vi "副屏设置.vi"() -> ()   [LabVIEW 2016, in "副屏.lvlib"]
uses:
  <vilib>/Utility/config.llb/NI_LVConfig.lvlib
panel:
  in  "启用副屏":bool=TRUE caption="氨氮禁用"
  in  "关闭":bool
  in  "底部状态栏显示信息":string="一体化微型水质监测系统"
  in  "流速":bool caption="氨氮禁用"
  in  "瞬时流量":bool caption="氨氮禁用"
  in  "湿度":bool=TRUE caption="氨氮禁用"
  in  "水位":bool caption="氨氮禁用"
  in  "室温":bool=TRUE caption="氨氮禁用"
  in  "CODCr":bool caption="氨氮禁用"
  in  "CODMn":bool caption="氨氮禁用"
  in  "总氮":bool caption="氨氮禁用"
  in  "总磷":bool caption="氨氮禁用"
  in  "氨氮":bool caption="氨氮禁用"
  in  "Turb":bool caption="氨氮禁用"
  in  "Cond":bool caption="氨氮禁用"
  in  "DO":bool caption="氨氮禁用"
  in  "pH":bool caption="氨氮禁用"
  in  "水温":bool caption="氨氮禁用"
  # "副屏显示信息设置"
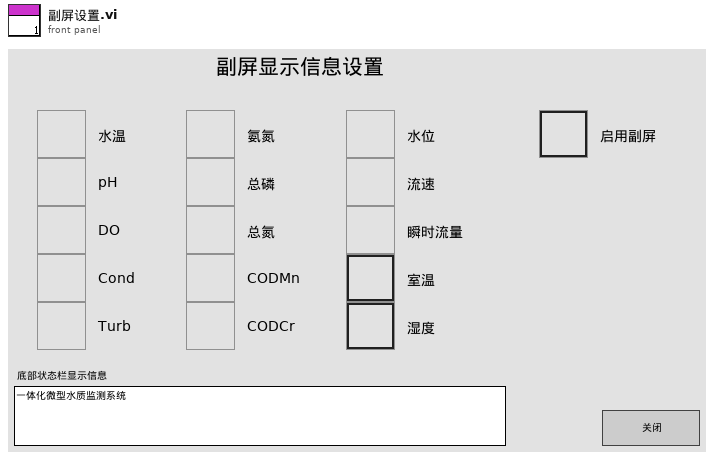
[diagram p1: front panel]
types:
  T1 = typedef "NI_LVConfig.lvlib/Config Data RefNum.ctl" = refnum<k1>
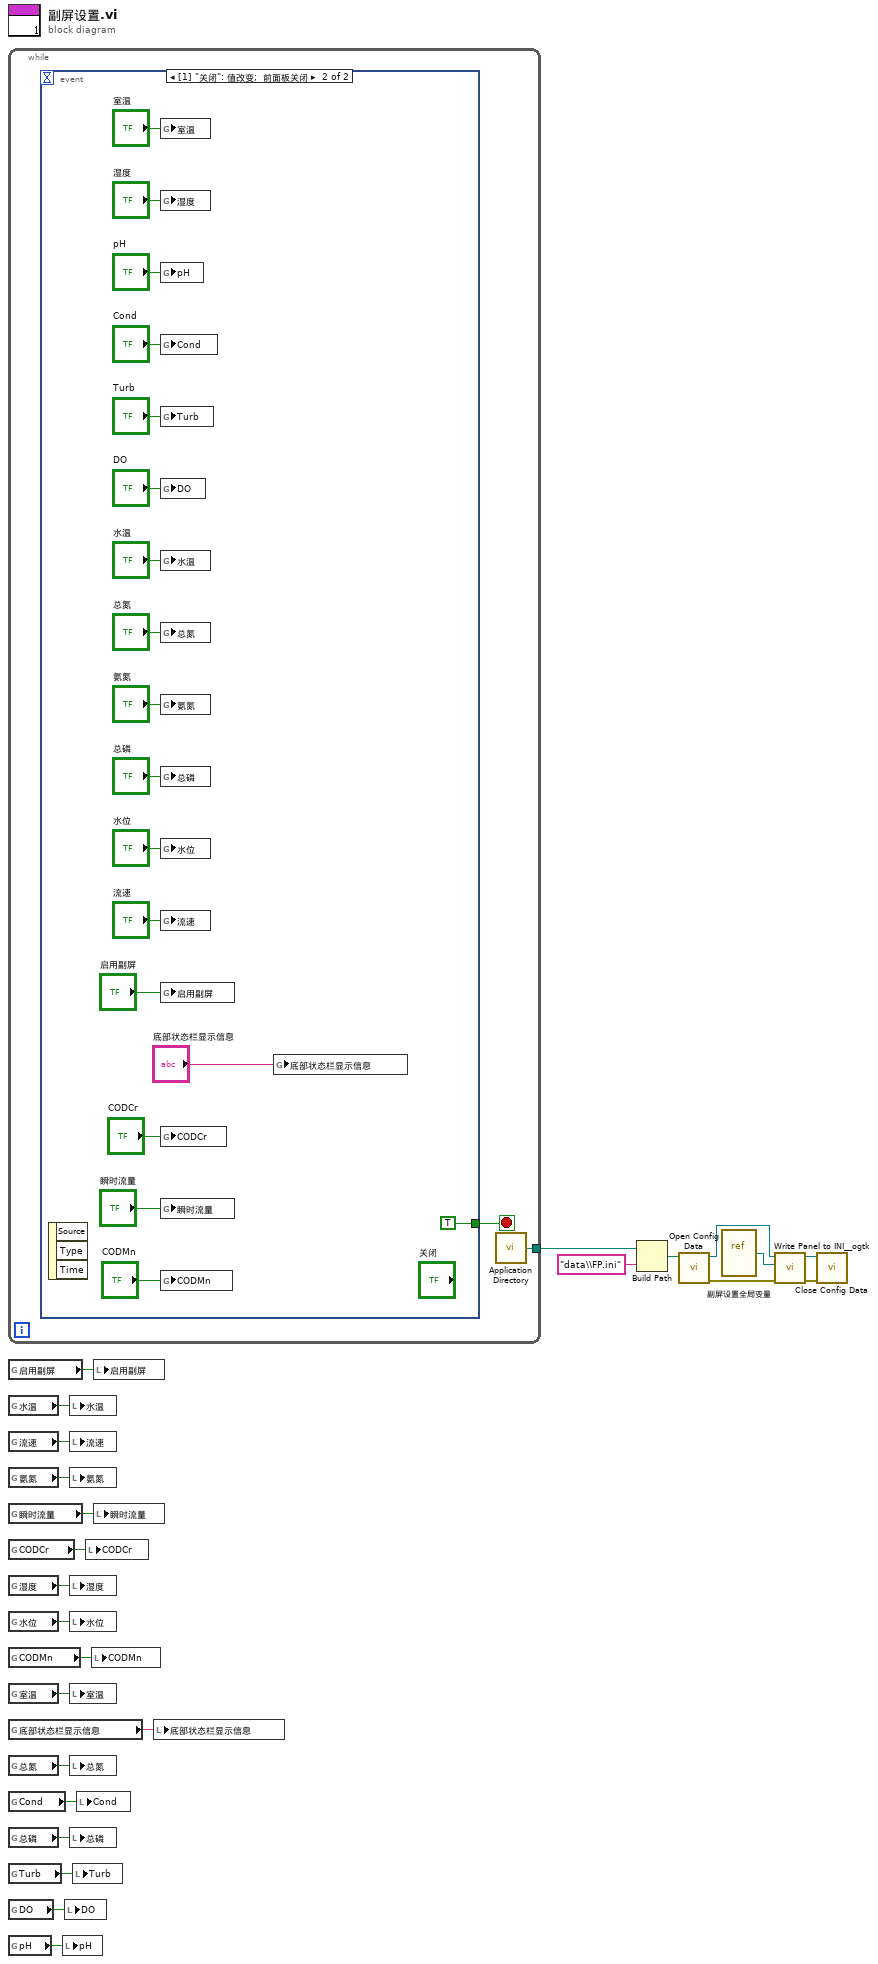
[diagram p0: block diagram]
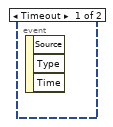
[diagram p2: hidden frame]
diagram:
  n1 = while {
    tunnel: [w26] -> w2
    stop <- w27 stop-if-true
    n2 = event shown="[1] \"关闭\": 值改变;  前面板关闭" {
      selector: _ -> [_ _]
      dyn-events: _ -> [_ _]
      timeout: _ -> [_ _]
      tunnel: [_ TRUE] -> w27
      event Timeout {
        n3 = event-data() -> ()  [unwired: 1 in, 3 out]
      }
      event "关闭": Value Change; Panel Close {
        n4 = event-data() -> ()  [unwired: 1 in, 3 out]
        n5 = global write "副屏设置全局变量.vi" "室温"("室温") -> ()
        n6 = global write "副屏设置全局变量.vi" "湿度"("湿度") -> ()
        n7 = global write "副屏设置全局变量.vi" "pH"("pH") -> ()
        n8 = global write "副屏设置全局变量.vi" "Cond"("Cond") -> ()
        n9 = global write "副屏设置全局变量.vi" "Turb"("Turb") -> ()
        n10 = global write "副屏设置全局变量.vi" "DO"("DO") -> ()
        n11 = global write "副屏设置全局变量.vi" "水温"("水温") -> ()
        n12 = global write "副屏设置全局变量.vi" "总氮"("总氮") -> ()
        n13 = global write "副屏设置全局变量.vi" "氨氮"("氨氮") -> ()
        n14 = global write "副屏设置全局变量.vi" "总磷"("总磷") -> ()
        n15 = global write "副屏设置全局变量.vi" "水位"("水位") -> ()
        n16 = global write "副屏设置全局变量.vi" "流速"("流速") -> ()
        n17 = global write "副屏设置全局变量.vi" "启用副屏"("启用副屏") -> ()
        n18 = global write "副屏设置全局变量.vi" "CODCr"("CODCr") -> ()
        n19 = global write "副屏设置全局变量.vi" "瞬时流量"("瞬时流量") -> ()
        n20 = global write "副屏设置全局变量.vi" "CODMn"("CODMn") -> ()
        n21 = global write "副屏设置全局变量.vi" "底部状态栏显示信息"("底部状态栏显示信息") -> ()
      }
    }
    n22 = call <vilib>:"Application Directory.vi"() -> ("Application Directory"=w26:path)
  }
  n23 = global read "副屏设置全局变量.vi" "启用副屏"() -> (w1:bool)
  n24 = global read "副屏设置全局变量.vi" "水温"() -> (w25:bool)
  n25 = global read "副屏设置全局变量.vi" "流速"() -> (w19:bool)
  n26 = global read "副屏设置全局变量.vi" "氨氮"() -> (w24:bool)
  n27 = global read "副屏设置全局变量.vi" "瞬时流量"() -> (w17:bool)
  n28 = global read "副屏设置全局变量.vi" "CODCr"() -> (w23:bool)
  n29 = global read "副屏设置全局变量.vi" "湿度"() -> (w16:bool)
  n30 = global read "副屏设置全局变量.vi" "水位"() -> (w22:bool)
  n31 = global read "副屏设置全局变量.vi" "CODMn"() -> (w21:bool)
  n32 = global read "副屏设置全局变量.vi" "室温"() -> (w13:bool)
  n33 = global read "副屏设置全局变量.vi" "底部状态栏显示信息"() -> (w20:string)
  n34 = global read "副屏设置全局变量.vi" "总氮"() -> (w14:bool)
  n35 = global read "副屏设置全局变量.vi" "Cond"() -> (w18:bool)
  n36 = global read "副屏设置全局变量.vi" "总磷"() -> (w11:bool)
  n37 = global read "副屏设置全局变量.vi" "Turb"() -> (w12:bool)
  n38 = global read "副屏设置全局变量.vi" "DO"() -> (w15:bool)
  n39 = global read "副屏设置全局变量.vi" "pH"() -> (w10:bool)
  n40 = local write "pH"(w10) -> ()
  n41 = local write "DO"(w15) -> ()
  n42 = local write "水温"(w25) -> ()
  n43 = local write "流速"(w19) -> ()
  n44 = local write "氨氮"(w24) -> ()
  n45 = local write "湿度"(w16) -> ()
  n46 = local write "水位"(w22) -> ()
  n47 = local write "室温"(w13) -> ()
  n48 = local write "总氮"(w14) -> ()
  n49 = local write "总磷"(w11) -> ()
  n50 = local write "Turb"(w12) -> ()
  n51 = local write "Cond"(w18) -> ()
  n52 = local write "CODCr"(w23) -> ()
  n53 = local write "CODMn"(w21) -> ()
  n54 = local write "启用副屏"(w1) -> ()
  n55 = local write "瞬时流量"(w17) -> ()
  n56 = local write "底部状态栏显示信息"(w20) -> ()
  n57 = Build Path(base path=w2, name or relative path="data\\FP.ini" ("名称或相对路径")) -> (appended path=w4:path)
  n58 = call <vilib>:"Open Config Data.vi"("configuration file path"=w4) -> ("error out"=w8:errorcluster, "refnum"=w5:T1)  [unwired: 8 in, 1 out]
  n59 = vi-ref "副屏设置全局变量.vi"() -> (w6:refnum<vi>)
  n60 = call <userlib>:"Write Panel to INI__ogtk.vi"("error in (no error)"=w8, "VI ref"=w6, "refnum"=w5) -> ("error out"=w9:errorcluster, "refnum out"=w7:T1)  [unwired: 7 in]
  n61 = call <vilib>:"Close Config Data.vi"("error in (no error)"=w9, "refnum"=w7) -> ()  [unwired: 8 in, 2 out]
